vi "Queue Receive.vi"(11 "Base Queue jettl in":refnum<class "Base Queue jettl.lvclass">) -> (2 "Msg Strategy":refnum<class "Msg Strategy.lvclass">, 3 "Base Queue jettl out":refnum<class "Base Queue jettl.lvclass">)   [LabVIEW 2021, in "jettl.lvlib" / "Base Queue jettl.lvlib" / "Base Queue jettl.lvclass"]
uses:
  Base Queue jettl.lvclass
  Msg Strategy/Msg Strategy.lvclass
  Base Queue jettl.lvclass/Base Queue jettl.ctl
  jettl.lvlib
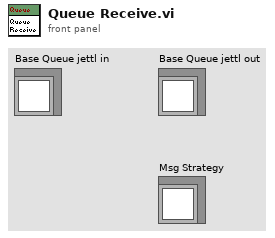
[diagram p1: front panel]
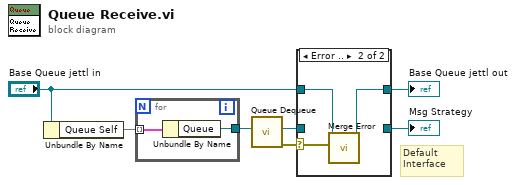
[diagram p0: block diagram]
diagram:
  # "Default Interface"
  n1 = Unbundle By Name("Base Queue jettl in") -> ("Queue Self"=w2:map{string, refnum<data-value>})
  n2 = for {
    tunnel: w2 -> [w9] mode=indexing
    tunnel: [w8] -> w1
    n3 = Unbundle By Name(w9) -> ("Queue"=w8:refnum<data-value>)
  }
  n4 = call "Queue Dequeue.vi"("Queue"=w1) -> ("error out"=w7:errorcluster, "Msg Strategy"=w6:refnum<class "Msg Strategy.lvclass">)  [unwired: 9 in]
  n5 = case shown="Error .." w7 {
    selector: w7 -> [_ w12]
    tunnel: w6 -> [w10 _]
    tunnel: "Base Queue jettl in" -> [w11 w14]
    tunnel: [w11 w13] -> w5
    tunnel: [w10 _] -> w4
    frame No Error {
    }
    frame Error {
      n6 = call-dynamic "Merge Error.vi"("Error"=w12, "Base Queue jettl in"=w14) -> ("Base Queue jettl out"=w13:refnum<class "Base Queue jettl.lvclass">)  [unwired: 9 in]
    }
  }
  "Base Queue jettl out" <- w5
  "Msg Strategy" <- w4
